vi "Get Enum String Items.vi"(7 "error in (no error)":errorcluster, 10 "Enum Refnum":refnum<vi>) -> (0 "error out":errorcluster, 2 "String":string)   [LabVIEW 2015]
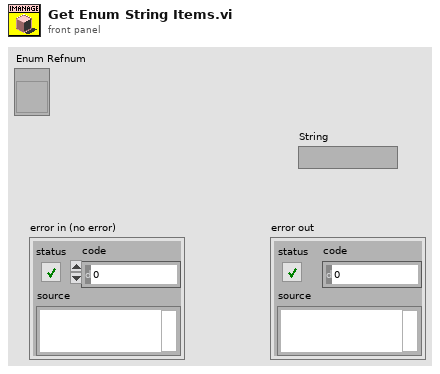
[diagram p1: front panel]
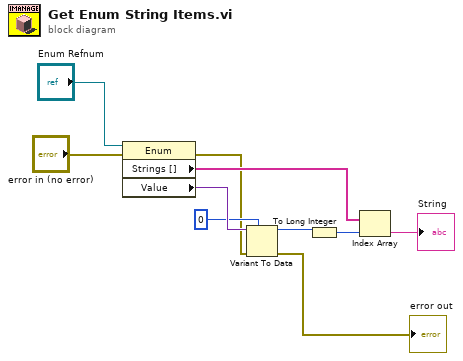
[diagram p0: block diagram]
diagram:
  n1 = property class="Enum"(reference="Enum Refnum", error in="error in (no error)") -> (error out=w2:errorcluster, "Strings []"=w9:string[], "Value"=w5:variant)  [unwired: 1 out]
  n2 = Variant To Data(error in=w2, type=u8 0, Variant=w5) -> (data=w3:u8, error out=→"error out":errorcluster)
  n3 = To Long Integer(number=w3) -> (32bit integer=w7:i32)
  n4 = Index Array(array=w9, index=w7) -> (element=→"String":string)
